vi "GOOP_MyComputer_Interface_CreateNewWizard_Interface.vi"() -> (3 "InterfaceTable":T1)   [LabVIEW 2020]
uses:
  <resource>/Framework/Providers/API/CreateNewWizard_Interface.ctl
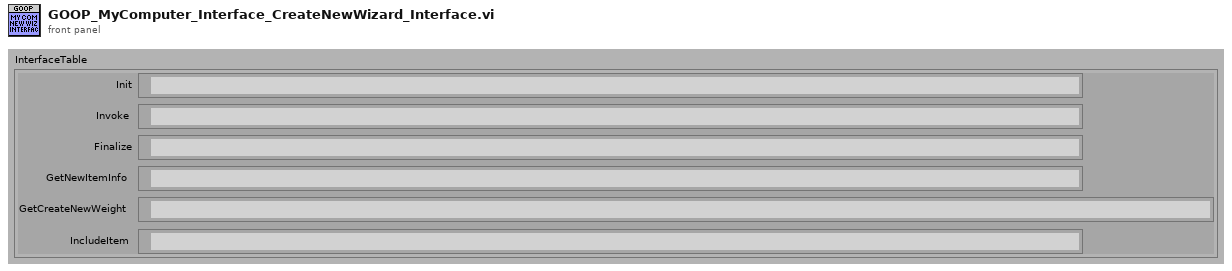
[diagram p1: front panel]
types:
  T1 = typedef "CreateNewWizard_Interface.ctl" = cluster{"Init":path, "Invoke":path, "Finalize":path, "GetNewItemInfo":path, "GetCreateNewWeight":path, "IncludeItem":path}
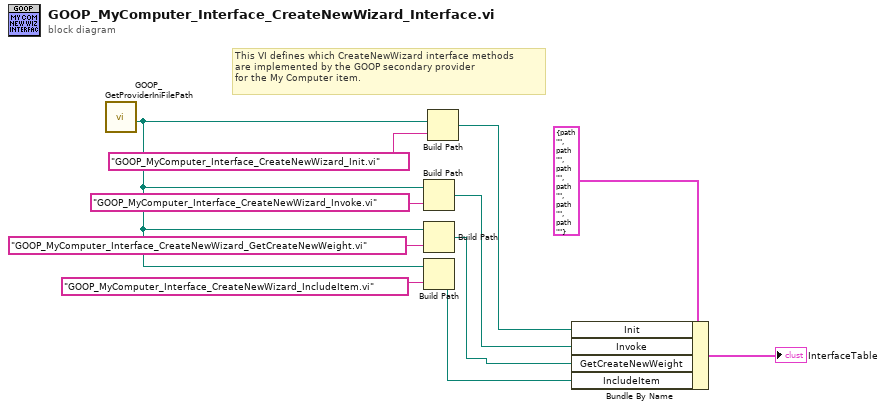
[diagram p0: block diagram]
diagram:
  # "This VI defines which CreateNewWizard interface methods \nare implemented by the GOOP secondary provider \nfor the My Computer item."
  n1 = call <resource>:"GOOP_GetProviderIniFilePath.vi"() -> ("ProviderMainFolder"=w6:path)  [unwired: 10 in, 1 out]
  n2 = Build Path(base path=w6, name or relative path="GOOP_MyComputer_Interface_CreateNewWizard_Invoke.vi") -> (appended path=w3:path)
  n3 = Build Path(base path=w6, name or relative path="GOOP_MyComputer_Interface_CreateNewWizard_GetCreateNewWeight.vi") -> (appended path=w2:path)
  n4 = Build Path(base path=w6, name or relative path="GOOP_MyComputer_Interface_CreateNewWizard_IncludeItem.vi") -> (appended path=w1:path)
  n5 = Build Path(base path=w6, name or relative path="GOOP_MyComputer_Interface_CreateNewWizard_Init.vi") -> (appended path=w4:path)
  n6 = Bundle By Name(cluster=T1 {"Init"=path "", "Invoke"=path "", "Finalize"=path "", "GetNewItemInfo"=path "", "GetCreateNewWeight"=path "", "IncludeItem"=path ""} ("InterfaceTable"), "Init"=w4, "Invoke"=w3, "GetCreateNewWeight"=w2, "IncludeItem"=w1) -> (→"InterfaceTable":T1)
